vi "Actor Core.vi"(8 "error in":errorcluster caption="错误输入", 11 "EPEVER-MPPT in":refnum<class "EPEVER-MPPT.lvclass"> caption="操作者输入") -> (0 "error out":errorcluster caption="错误输出", 3 "Actor out":refnum<class "Actor.lvclass"> caption="操作者输出")   [LabVIEW 2016, in "EPEVER-MPPT.lvlib" / "EPEVER-MPPT.lvclass"]
doc: "(<B>Filename</B>: Actor Framework.lvlib:Actor.lvclass:Actor Core.vi)\n\nReceives messages to the actor, reacts to them, and initiates any error handling that may shut the actor down.\n\nDescendant classes may override this VI to append parallel tasks for the actor to complete while it handles messages.使用调用父方法节点实现重写。"
uses:
  EPEVER-MPPT.lvclass
  C:/Program Files (x86)/National Instruments/LabVIEW 2016/vi.lib/ActorFramework/Actor/Actor.lvclass
  <vilib>/ActorFramework/Actor/Actor.lvclass
  <vilib>/ActorFramework/Actor/Actor.lvclass/Actor.ctl
  <vilib>/ActorFramework/Message Enqueuer/Message Enqueuer.lvclass/Message Enqueuer.ctl
  <vilib>/ActorFramework/Message Enqueuer/Init from Existing Queue.vi
  <vilib>/ActorFramework/Message Enqueuer/Enqueue.vi
  C:/Program Files (x86)/National Instruments/LabVIEW 2016/vi.lib/ActorFramework/Message/Message.lvclass
  <vilib>/ActorFramework/Message Priority Queue/Priority Enqueue.vi
  <vilib>/ActorFramework/Message Enqueuer/Message Enqueuer.lvclass
panel:
  in  "布尔":bool
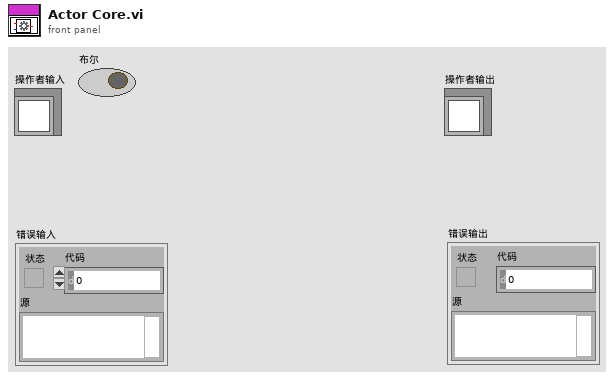
[diagram p1: front panel]
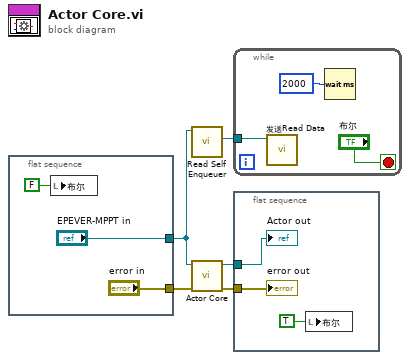
[diagram p0: block diagram]
diagram:
  n1 = flat-sequence {
    tunnel: ["error in"] -> w3
    tunnel: ["EPEVER-MPPT in"] -> w2
    frame #0 {
      n2 = local write "布尔"(FALSE ("布尔")) -> ()
    }
  }
  n3 = call <vilib>:"Read Self Enqueuer.vi"("Actor"=w2) -> ("Self Enqueuer"=w1:refnum<class "Message Enqueuer.lvclass">)  [unwired: 10 in]
  n4 = call-parent "Actor Core.vi"("error in"=w3, "Actor in"=w2) -> ("error out"=w5:errorcluster, "Actor out"=w4:refnum<class "Actor.lvclass">)  [unwired: 8 in]
  n5 = while {
    tunnel: w1 -> [w10]
    stop <- "布尔" stop-if-true
    n6 = call "发送Read Data.vi"("Message Enqueuer"=w10) -> ()  [unwired: 9 in, 2 out]
    n7 = Wait (ms)(milliseconds to wait=u32 2000 ("等待时间（毫秒）")) -> ()  [unwired: 1 out]
  }
  n8 = flat-sequence {
    tunnel: w5 -> [w14]
    tunnel: w4 -> [w13]
    frame #0 {
      n9 = local write "布尔"(TRUE ("布尔")) -> ()
      "error out" <- w14
      "Actor out" <- w13
    }
  }
